vi "TDMS - Perform RT Data Portion.vi"(8 "error in (no error)":errorcluster, 11 "View Model":T1) -> (0 "error out":errorcluster, 1 "Not Empty?":bool, 2 "2D RT Data Portion":dbl[][](array[numeric]), 3 "View Model":T1)   [LabVIEW 2017]
doc: "SubVI Perform a portion of RT Data for saving"
uses:
  View Model/Controls/View Model.ctl
  View Model/Controls/Shared Model.ctl
  Error Handler/Controls/Error Model.ctl
  Error Handler/Controls/Error Event.ctl
  Error Handler/Controls/Error Type.ctl
  Controller/Controls/Controller Model.ctl
  Controller/Controls/Controller Event.ctl
  Controller/Controls/Controller Command.ctl
  Controller/Controls/Controller Overhead.ctl
  Real-Time/RT Status.ctl
  Real-Time/RT Loop Status.ctl
  Controller/Controls/Controller NStream.ctl
  Controller/Controls/Controller Timer Data.ctl
  Controller/Controls/Controller DAQ Data.ctl
  Controls/TDMS Model.ctl
  Controls/TDMS Event.ctl
  Controls/TDMS Command.ctl
  Controls/TDMS Overhead.ctl
  Controls/TDMS ChanProperties.ctl
  Controls/TDMS DAQ Data.ctl
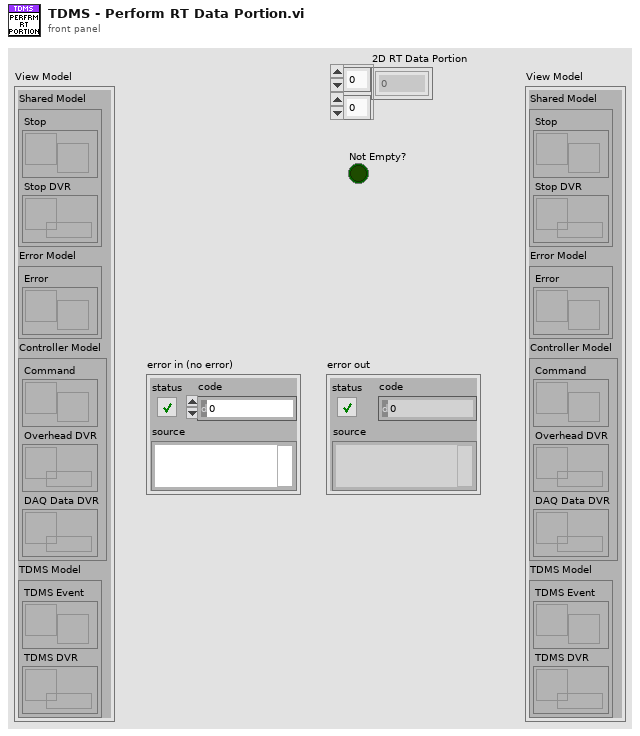
[diagram p1: front panel]
types:
  T1 = typedef "View Model.ctl" = cluster{"Shared Model":T2, "Error Model":T3, "Controller Model":T4, "TDMS Model":T5}
  T2 = typedef "Shared Model.ctl" = cluster{"Stop":refnum<user-event>, "Stop DVR":refnum<data-value>}
  T3 = typedef "Error Model.ctl" = cluster{"Error":refnum<user-event>}
  T4 = typedef "Controller Model.ctl" = cluster{"Command":refnum<user-event>, "Overhead DVR":refnum<data-value>, "DAQ Data DVR":refnum<data-value>}
  T5 = typedef "TDMS Model.ctl" = cluster{"TDMS Event":refnum<user-event>, "TDMS DVR":refnum<data-value>}
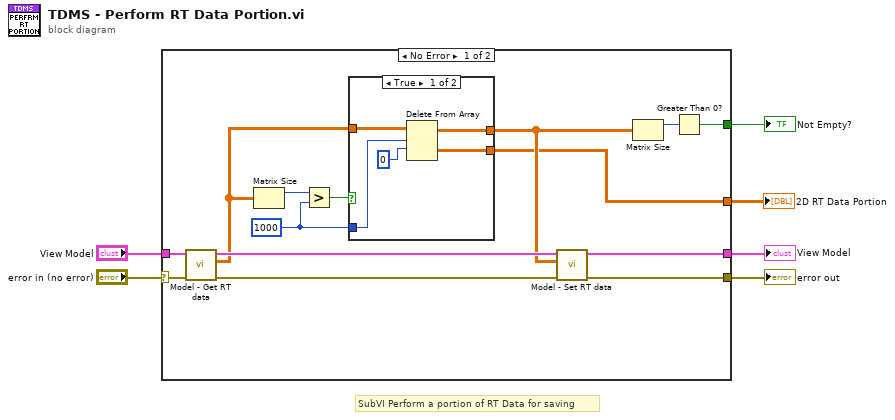
[diagram p0: block diagram]
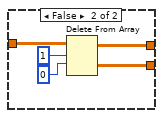
[diagram p2: hidden frame]
diagram:
  # "SubVI Perform a portion of RT Data for saving"
  n1 = case shown="No Error" "error in (no error)" {
    selector: "error in (no error)" -> [w15 w31]
    tunnel: [w12 w31] -> w5
    tunnel: "View Model" -> [w16 w32]
    tunnel: [w13 w32] -> w3
    tunnel: [w14 _] -> w2
    tunnel: [w11 _] -> w1
    frame No Error {
      w7 = 1000 ("y")
      n2 = call "Model - Get RT data.vi"("error in (no error)"=w15, "View Model"=w16) -> ("error out"=w19:errorcluster, "RT data"=w10:dbl[][], "View Model"=w20:T1)  [unwired: 7 in]
      n3 = Matrix Size(0:w10) -> (1:w9:i32)  [unwired: 1 out]
      n4 = Greater?(x=w9, y=w7) -> (0:w8:bool)
      n5 = case shown="True" w8 {
        tunnel: [w24 w28] -> w17
        tunnel: [w23 w27] -> w11
        tunnel: w10 -> [w22 w26]
        tunnel: w7 -> [w21 _]
        frame True {
          n6 = Delete From Array "Delete From Array"(array=w22, length=w21, index (row)=0) -> (deleted portion=w23:dbl[][], array with subset deleted=w24:dbl[][])  [unwired: 1 in]
        }
        frame False {
          n7 = Delete From Array "Delete From Array"(array=w26, length=1, index (row)=0) -> (deleted portion=w27:dbl[][], array with subset deleted=w28:dbl[][])  [unwired: 1 in]
        }
      }
      n8 = call "Model - Set RT data.vi"("error in (no error)"=w19, "RT data"=w17, "View Model"=w20) -> ("error out"=w12:errorcluster, "View Model"=w13:T1)  [unwired: 7 in]
      n9 = Matrix Size(0:w17) -> (1:w18:i32)  [unwired: 1 out]
      n10 = Greater Than 0?(x=w18) -> (x > 0?=w14:bool)
    }
    frame Error {
    }
  }
  "View Model" <- w3
  "error out" <- w5
  "Not Empty?" <- w2
  "2D RT Data Portion" <- w1
